vi "HEXISTS.vi"(8 "error in (no error)":errorcluster, 9 "field":string, 10 "key":string, 11 "Redis Client in":refnum<class "Redis Client.lvclass">) -> (0 "error out":errorcluster, 2 "exists?":bool, 3 "Redis Client out":refnum<class "Redis Client.lvclass">)   [LabVIEW 2019, in "Redis Client for LabVIEW.lvlib" / "Redis Client.lvclass"]
uses:
  Redis Client.lvclass
  RESP3 for LabVIEW/RESP3/high-level/RESP3 Make Bulk String.vi
  RESP3 for LabVIEW/RESP3/high-level/RESP3 Get Integer.vi
  RESP3 for LabVIEW/RESP3/RESP3.lvlib
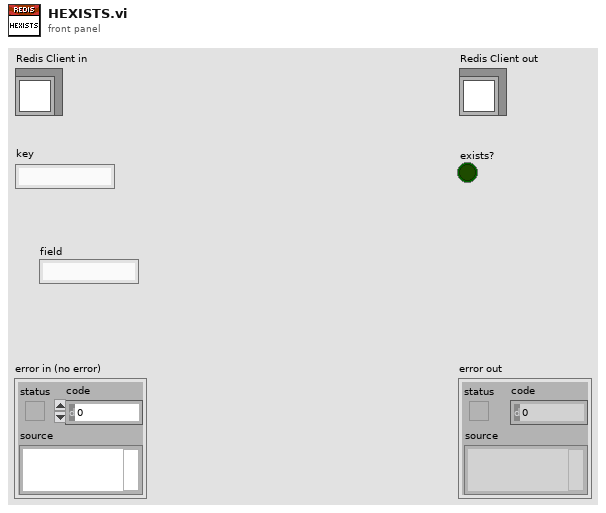
[diagram p1: front panel]
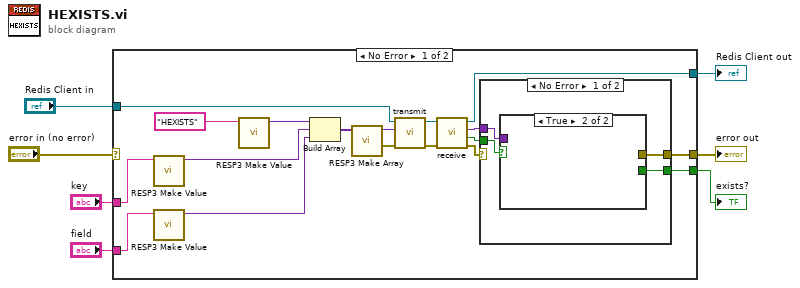
[diagram p0: block diagram]
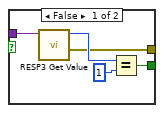
[diagram p2: hidden frame]
diagram:
  n1 = case shown="No Error" "error in (no error)" {
    selector: "error in (no error)" -> [_ w37]
    tunnel: [w22 w37] -> w6
    tunnel: "Redis Client in" -> [w25 w36]
    tunnel: [w24 w36] -> w4
    tunnel: "key" -> [w13 _]
    tunnel: "field" -> [w15 _]
    tunnel: [w23 _] -> w1
    frame No Error {
      n2 = call-poly "RESP3 Make Value.vi"("String"=w13) -> ("RESP3 Value out"=w12:variant)  [unwired: 9 in, 1 out]
      n3 = call-poly "RESP3 Make Value.vi"("String"=w15) -> ("RESP3 Value out"=w14:variant)  [unwired: 9 in, 1 out]
      n4 = call-poly "RESP3 Make Value.vi"("String"="HEXISTS" ("string in")) -> ("RESP3 Value out"=w10:variant)  [unwired: 9 in, 1 out]
      n5 = Build Array(w10, w12, w14) -> (w21:variant[])
      n6 = call "RESP3 Make Array.vi"("RESP3 Values in"=w21) -> ("error out"=w9:errorcluster, "RESP3 Value out"=w8:variant)  [unwired: 9 in]
      n7 = call-dynamic "transmit.vi"("error in (no error)"=w9, "RESP3 Value"=w8, "Redis Client in"=w25) -> ("error out"=w19:errorcluster, "Redis Client out"=w20:refnum<class "Redis Client.lvclass">)  [unwired: 7 in]
      n8 = call-dynamic "receive.vi"("error in (no error)"=w19, "Redis Client in"=w20) -> ("error out"=w16:errorcluster, "timed out?"=w17:bool, "RESP3 Value"=w18:variant, "Redis Client out"=w24:refnum<class "Redis Client.lvclass">)  [unwired: 6 in]
      n9 = case shown="No Error" w16 {
        selector: w16 -> [_ w35]
        tunnel: [w29 _] -> w23
        tunnel: [w28 w35] -> w22
        tunnel: w18 -> [w27 _]
        tunnel: w17 -> [w26 _]
        frame No Error {
          n10 = case shown="True" w26 {
            tunnel: [w31 _] -> w29
            tunnel: [w30 _] -> w28
            tunnel: w27 -> [w34 _]
            frame False {
              n11 = call-poly "RESP3 Get Value.vi"("RESP3 Value in"=w34) -> ("error out"=w30:errorcluster, "I64 out"=w33:i64)  [unwired: 8 in, 1 out]
              n12 = Equal?(x=w33, y=i64 1) -> (x = y?=w31:bool)
            }
            frame True {
            }
          }
        }
        frame Error {
        }
      }
    }
    frame Error {
    }
  }
  "error out" <- w6
  "Redis Client out" <- w4
  "exists?" <- w1
